vi "GetParam.vi"(8 "error in (no error)":errorcluster caption="entrée d'erreur (pas d'erreur)", 11 "Johnson_lindenstrauss_min_dim.lvclass":refnum<class "Johnson_lindenstrauss_min_dim.lvclass">) -> (0 "error out":errorcluster caption="sortie d'erreur", 2 "johnson_lindenstrauss_min_dim":cluster{"n_samples":i32[], "eps":dbl[]} {"eps" min=0.0 max=1.0}, 3 "Johnson_lindenstrauss_min_dim.lvclass":refnum<class "Johnson_lindenstrauss_min_dim.lvclass">)   [LabVIEW 2020, in "Johnson_lindenstrauss_min_dim.lvclass"]
doc: "Get Parameters"
uses:
  Johnson_lindenstrauss_min_dim.lvclass
  Johnson_lindenstrauss_min_dim.lvclass/Johnson_lindenstrauss_min_dim.ctl
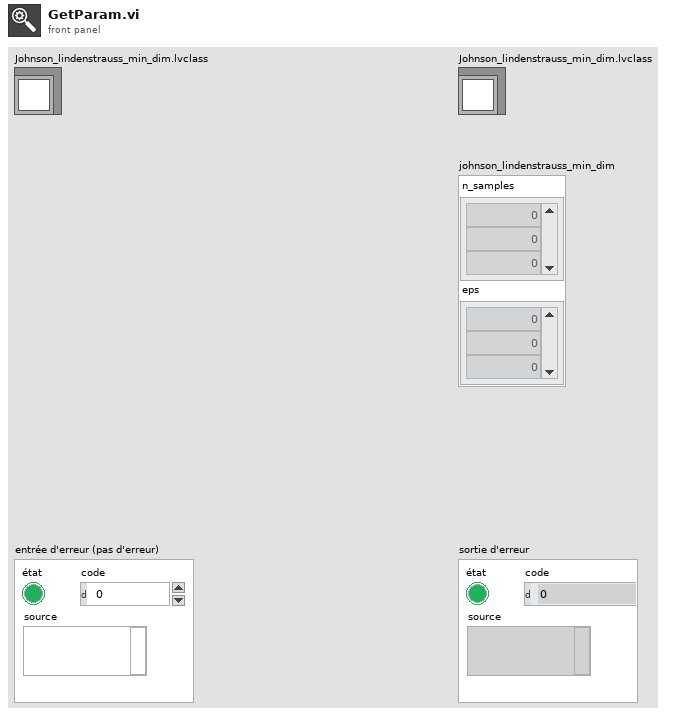
[diagram p1: front panel]
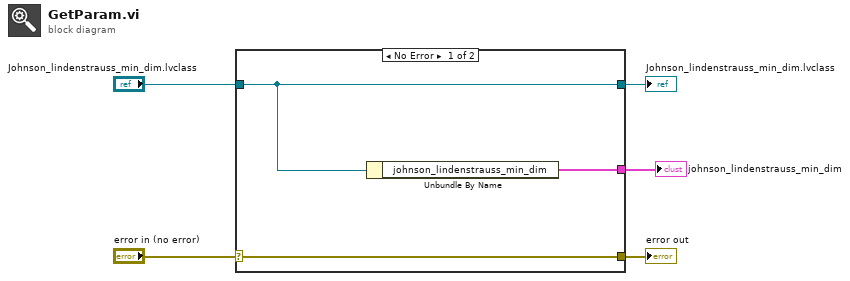
[diagram p0: block diagram]
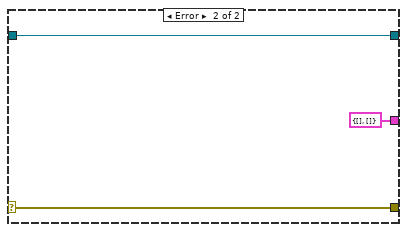
[diagram p2: hidden frame]
diagram:
  n1 = case shown="No Error" "error in (no error)" {
    selector: "error in (no error)" -> [w8 w10]
    tunnel: [w8 w10] -> w4
    tunnel: [w7 w11] -> w2
    tunnel: "Johnson_lindenstrauss_min_dim.lvclass" -> [w7 w11]
    tunnel: [w6 cluster{"n_samples":i32[], "eps":dbl[]} {"n_samples"=[], "eps"=[]} ("johnson_lindenstrauss_min_dim")] -> w1
    frame No Error {
      n2 = Unbundle By Name(w7) -> ("johnson_lindenstrauss_min_dim"=w6:cluster{"n_samples":i32[], "eps":dbl[]})
    }
    frame Error {
    }
  }
  "error out" <- w4
  "Johnson_lindenstrauss_min_dim.lvclass" <- w2
  "johnson_lindenstrauss_min_dim" <- w1
